vi "partial_fit.vi"(8 "error in (no error)":errorcluster caption="entrée d'erreur (pas d'erreur)", 11 "LatentDirichletAllocation.lvclass 2":refnum<class "LatentDirichletAllocation.lvclass">) -> (0 "error out":errorcluster caption="sortie d'erreur", 3 "LatentDirichletAllocation.lvclass":refnum<class "LatentDirichletAllocation.lvclass">)   [LabVIEW 2020, in "LatentDirichletAllocation.lvclass"]
doc: "Online VB with Mini-Batch update."
uses:
  LatentDirichletAllocation.lvclass
  C:/Users/cipop/TDF Dropbox/2_Technologies de France/1 - Services et Etudes/PLAIY/2 - DEV/PLAIYLAB/code/Python/Python.lvclass
  C:/Users/cipop/TDF Dropbox/2_Technologies de France/1 - Services et Etudes/PLAIY/2 - DEV/PLAIYLAB/code/Model/Model.lvclass
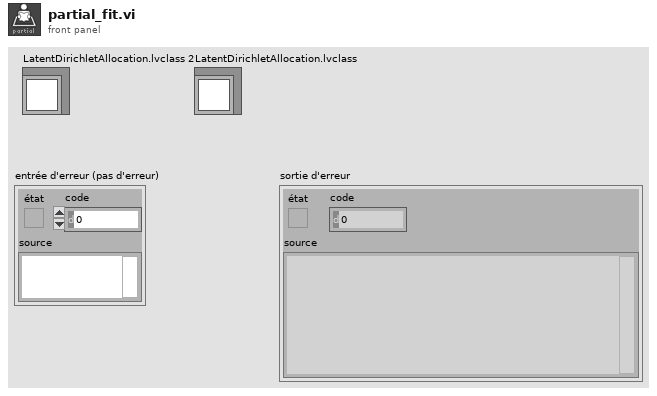
[diagram p1: front panel]
types:
  T1 = typedef "data.ctl" = cluster{"name":string, "X":dbl[][]}
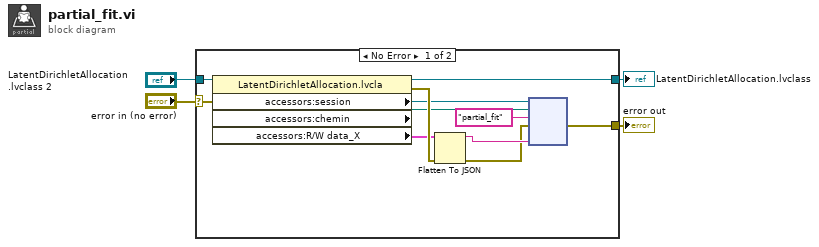
[diagram p0: block diagram]
diagram:
  n1 = case shown="No Error" "error in (no error)" {
    selector: "error in (no error)" -> [w13 w17]
    tunnel: [w14 w17] -> w3
    tunnel: [w6 w16] -> w1
    tunnel: "LatentDirichletAllocation.lvclass 2" -> [w5 w16]
    frame No Error {
      n2 = property class="LatentDirichletAllocation.lvcla"(reference=w5, error in=w13) -> (reference out=w6:refnum<class "LatentDirichletAllocation.lvclass">, error out=w11:errorcluster, "accessors:session"=w8:refnum<k35>, "accessors:chemin"=w7:path, "accessors:R/W data_X"=w9:T1)
      n3 = Flatten To JSON(anything=w9, error in (no error)=w11) -> (JSON string=w12:string, 11:w10:errorcluster)  [unwired: 1 in]
      n4 = node(w8, w7, "partial_fit" ("nom de la fonction"), w10, w12) -> (w14:errorcluster)  [unwired: 3 in, 3 out]
    }
    frame Error {
    }
  }
  "error out" <- w3
  "LatentDirichletAllocation.lvclass" <- w1
